vi "Check Accessories Busy.vi"(8 "error in (no error)":errorcluster, 11 "VISA resource name":refnum<visa-resource-name>) -> (0 "error out":errorcluster, 2 "busy?":bool, 3 "VISA resource name out":refnum<visa-resource-name>)   [LabVIEW 2009, in "JY-SPEX-TRIAX.lvlib"]
doc: "Used to poll the accessories (turret, mirrors, shutter) after moving them. Unlike with the motor and slits, multiple accessories can be moved at the same time. This VI is most useful to check and make sure that all accessories have finished moving before beginning an acquisition."
uses:
  JY-SPEX-TRIAX.lvlib
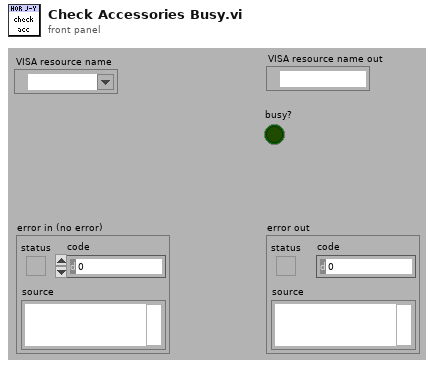
[diagram p1: front panel]
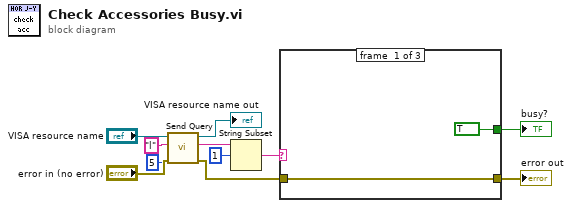
[diagram p0: block diagram]
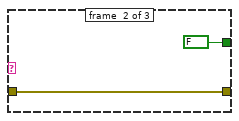
[diagram p2: hidden frame]
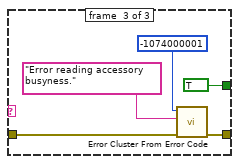
[diagram p3: hidden frame]
diagram:
  n1 = call "Send Query.vi"("error in (no error)"="error in (no error)", "byte count"=u32 5, "write buffer"="l", "VISA resource name"="VISA resource name") -> ("error out"=w4:errorcluster, "read buffer"=w7:string, "VISA resource name out"=→"VISA resource name out":refnum<visa-resource-name>)  [unwired: 5 out]
  n2 = String Subset(string=w7, offset (0)=1) -> (substring=w5:string)  [unwired: 1 out]
  n3 = case shown="Default" w5 {
    tunnel: w4 -> [w13 w15 w17]
    tunnel: [w13 w15 w18] -> w2
    tunnel: [TRUE FALSE TRUE] -> w1
    frame #0 {
    }
    frame #1 {
    }
    frame #2 {
      n4 = call <vilib>:"Error Cluster From Error Code.vi"("error in (no error)"=w17, "error message (\"\")"="Error reading accessory busyness." ("error message (\"\")"), "error code (0)"=-1074000001) -> ("error out"=w18:errorcluster)  [unwired: 1 in, 5 out]
    }
  }
  "busy?" <- w1
  "error out" <- w2
